vi "ziModGetNodeValueString.vi"(0 "ModHandle In":T1 {"ModHandle" format="0x%08x"; "Conn" format="0x%08x"}, 7 "Path":string, 11 "error in":errorcluster) -> (4 "ModHandle Out":T1 {"ModHandle" format="0x%08x"; "Conn" format="0x%08x"}, 8 "Value":string, 15 "error out":errorcluster)   [LabVIEW 2018, in "Zurich Instruments LabOne.lvlib"]
doc: "FOR MODULES This vi retrieves the value of the node node specified by <b>Path</b> as a string <b>value</b>. The vi returns the value of the node first found if more than one node is available (a wildcard is used in <b>Path</b>). This function is only applicable to nodes that contain strings."
uses:
  Zurich Instruments LabOne.lvlib
  ziTypeModHandle.ctl
  ziLV32.dll
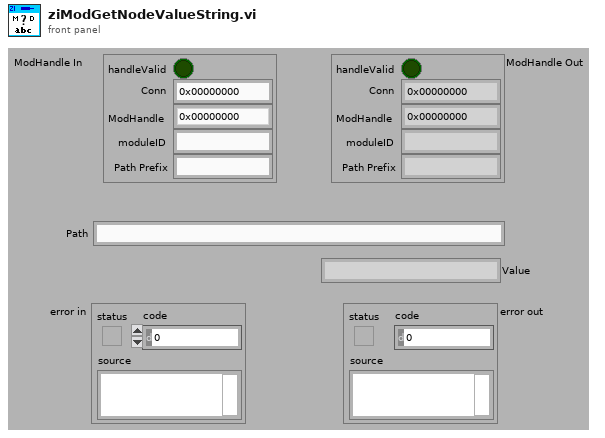
[diagram p1: front panel]
types:
  T1 = typedef "Zurich Instruments LabOne.lvlib/ziTypeModHandle.ctl" = cluster{"handleValid":bool, "Conn":u64, "ModHandle":u64, "moduleID":string, "Path Prefix":string}
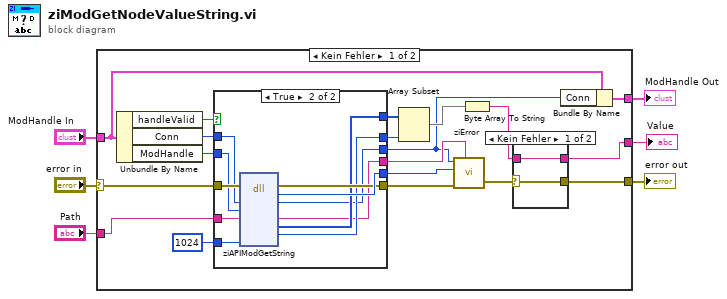
[diagram p0: block diagram]
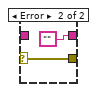
[diagram p2: hidden frame]
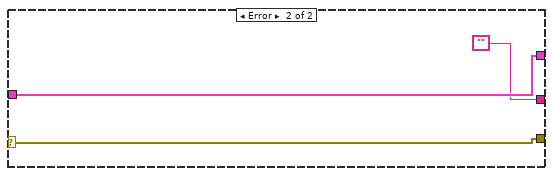
[diagram p4: hidden frame]
diagram:
  n1 = case shown="Kein Fehler" "error in" {
    selector: "error in" -> [w18 w46]
    tunnel: [w8 w46] -> w6
    tunnel: [w23 w45] -> w1
    tunnel: "ModHandle In" -> [w13 w45]
    tunnel: "Path" -> [w14 _]
    tunnel: [w7 ""] -> w4
    frame No Error {
      n2 = Unbundle By Name(w13) -> ("handleValid"=w11:bool, "Conn"=w16:u64, "ModHandle"=w12:u64)
      n3 = case shown="True" w11 {
        tunnel: [_ w43] -> w25
        tunnel: [w32 w42] -> w24
        tunnel: 1024 ("MaxLen") -> [_ w41]
        tunnel: [_ w40] -> w21
        tunnel: [_ w39] -> w20
        tunnel: w18 -> [w32 w38]
        tunnel: [w30 w37] -> w17
        tunnel: w16 -> [w31 w36]
        tunnel: [w31 w35] -> w15
        tunnel: w14 -> [w30 w34]
        tunnel: w12 -> [_ w33]
        frame False {
        }
        frame True {
          n4 = dll-call lib="ziLV*.*" fn="ziAPIModGetString"(error in=w38, "Conn"=w36, "ModHandle"=w33, "Path"=w34, "MaxLen"=w41) -> (error out=w42:errorcluster, "return type"=w43:u32, "Conn"=w35:u64, "Path"=w37:string, "Buffer"=w40:i8[], "Len"=w39:i32)  [unwired: 3 in, 4 out]
        }
      }
      n5 = Array Subset(array=w21, length=w20) -> (w19:i8[])  [unwired: 1 in]
      n6 = call "ziError.vi"("Conn"=w15, "ziErrorCode"=w25, "Error In"=w24, "Annotation"=w17) -> ("Error Out"=w9:errorcluster)  [unwired: 2 in]
      n7 = Byte Array To String(unsigned byte array=w19) -> (string=w10:string)
      n8 = case shown="Kein Fehler" w9 {
        selector: w9 -> [w27 w29]
        tunnel: w10 -> [w26 _]
        tunnel: [w27 w29] -> w8
        tunnel: [w26 ""] -> w7
        frame No Error {
        }
        frame Error {
        }
      }
      n9 = Bundle By Name(cluster=w13, "Conn"=w15) -> (w23:T1)
    }
    frame Error {
    }
  }
  "error out" <- w6
  "Value" <- w4
  "ModHandle Out" <- w1
